vi "Dialog Button.vi"   [LabVIEW 2018]
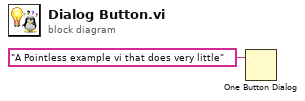
[diagram p0: block diagram]
diagram:
  n1 = One Button Dialog(message="A Pointless example vi that does very little") -> ()  [unwired: 1 in, 1 out]
